vi "Get LabVIEW Server ID.vi"(7 "Server Alias":string, 10 "Error In":errorcluster) -> (2 "Error Out":errorcluster, 3 "LabVIEW Server ID":string)   [LabVIEW 2013, in "TS.lvlib"]
uses:
  TS.lvlib
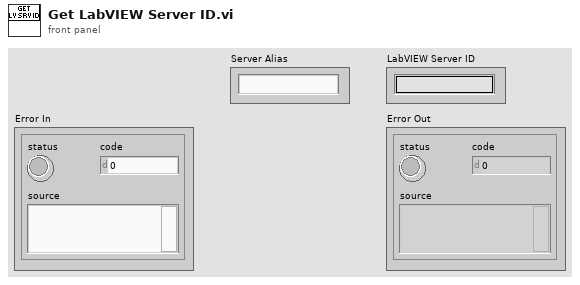
[diagram p1: front panel]
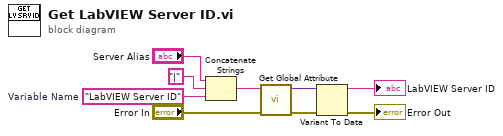
[diagram p0: block diagram]
diagram:
  w2 = "LabVIEW Server ID"  # Variable Name
  n1 = Concatenate Strings("Server Alias", "|" ("string"), w2) -> (w1:string)
  n2 = call "Get Global Attribute.vi"("Error In"="Error In", "Name"=w1) -> ("Error Out"=w9:errorcluster, "Value"=w8:variant)  [unwired: 7 in, 1 out]
  n3 = Variant To Data(error in=w9, Variant=w8) -> (data=→"LabVIEW Server ID":string, error out=→"Error Out":errorcluster)  [unwired: 1 in]
